vi "Write Player Info.vi"(8 "error in (no error)":errorcluster, 10 "Player Info":T1={"Name"="", "Color Box"=0, "Gloat Phrase"="All your base are belong to us!!"}, 11 "Wanderer in":refnum<class "Wanderer.lvclass">) -> (0 "error out":errorcluster, 3 "Wanderer out":refnum<class "Wanderer.lvclass">)   [LabVIEW 2014, in "Wanderer.lvclass"]
uses:
  Wanderer.lvclass
  Player Info.ctl
  Square.lvclass
  SquareBattle Arena/SquareBattle Arena.lvclass
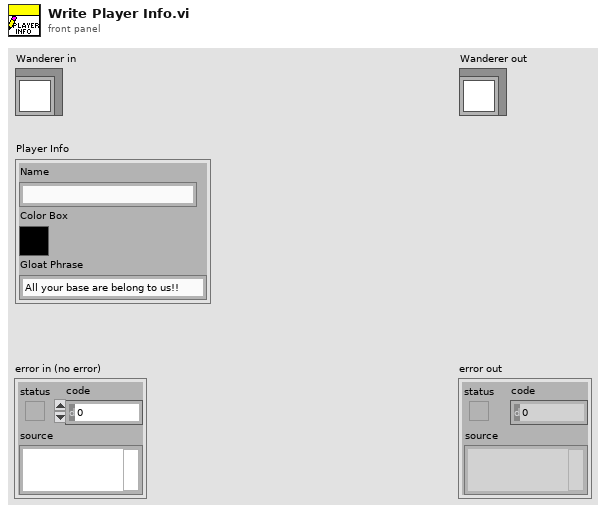
[diagram p1: front panel]
types:
  T1 = typedef "SquareBattle Arena.lvlib/SquareBattle Arena.lvclass/Player Info.ctl" = cluster{"Name":string, "Color Box":u32, "Gloat Phrase":string}
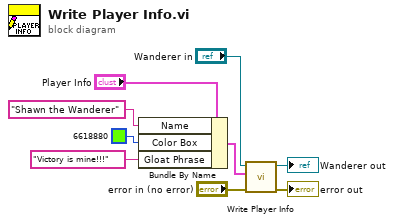
[diagram p0: block diagram]
diagram:
  n1 = Bundle By Name(cluster="Player Info", "Name"="Shawn the Wanderer", "Color Box"=u32 6618880, "Gloat Phrase"="Victory is mine!!!") -> (w4:T1)
  n2 = call-parent "Write Player Info.vi"("error in (no error)"="error in (no error)", "Player Info"=w4, "Runner in"="Wanderer in") -> ("error out"=→"error out":errorcluster, "Runner out"=→"Wanderer out":refnum<class "Wanderer.lvclass">)  [unwired: 7 in]
